vi "Post VI Refnum.vi"(8 "error in (no error)":errorcluster, 11 "Controller Template in":refnum<class "DemoCameraController.lvclass">) -> (0 "error out":errorcluster, 3 "Controller Template out":refnum<class "DemoCameraController.lvclass">)   [LabVIEW 2020, in "DemoCameraController.lvlib" / "DemoCameraController.lvclass"]
uses:
  DemoCameraController.lvclass
  C:/Program Files/National Instruments/LabVIEW 2020/vi.lib/ActorFramework/Actor/Actor.lvclass
  <vilib>/ActorFramework/Actor/Actor.lvclass/Actor.ctl
  DemoCameraController.lvclass/DemoCameraController.ctl
  Model/Hardware Abstraction Layer/Component/Device/Device Messages/Post VI Refnum Msg/Post VI Refnum Msg.lvclass/Post VI Refnum Msg.ctl
  <vilib>/ActorFramework/Message Enqueuer/Message Enqueuer.lvclass/Message Enqueuer.ctl
  <vilib>/ActorFramework/Message Enqueuer/Enqueue.vi
  Model/Hardware Abstraction Layer/Component/Device/Device Messages/Post VI Refnum Msg/Post VI Refnum Msg.lvclass
  C:/Program Files/National Instruments/LabVIEW 2020/vi.lib/ActorFramework/Message/Message.lvclass
  <vilib>/ActorFramework/Message Priority Queue/Priority Enqueue.vi
  <vilib>/ActorFramework/Actor/Actor.lvclass
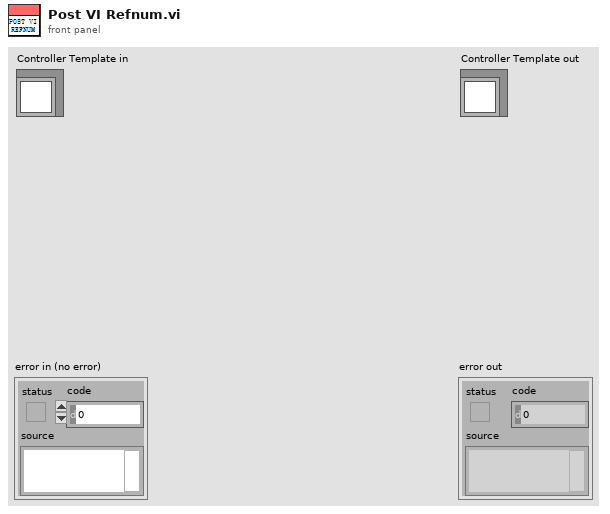
[diagram p1: front panel]
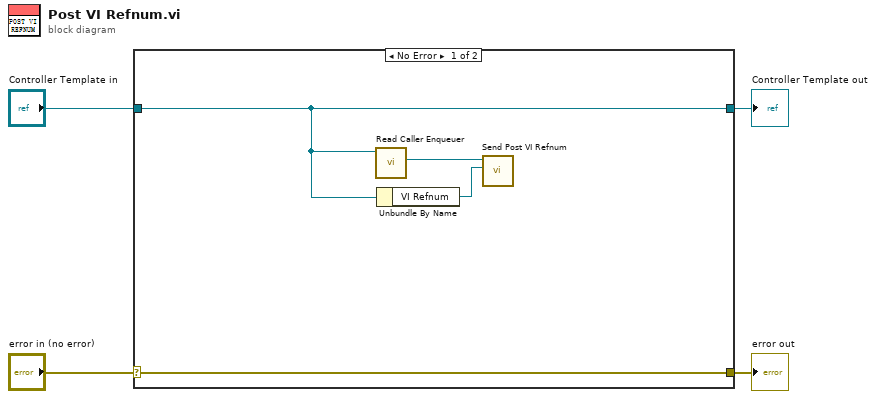
[diagram p0: block diagram]
diagram:
  n1 = case shown="No Error" "error in (no error)" {
    selector: "error in (no error)" -> [w8 w10]
    tunnel: [w8 w10] -> w3
    tunnel: [w5 w9] -> w1
    tunnel: "Controller Template in" -> [w5 w9]
    frame No Error {
      n2 = call <vilib>:"Read Caller Enqueuer.vi"("Actor"=w5) -> ("Caller Enqueuer"=w7:refnum<class "Message Enqueuer.lvclass">)  [unwired: 10 in]
      n3 = Unbundle By Name(w5) -> ("VI Refnum"=w6:refnum<vi>)
      n4 = call "Send Post VI Refnum.vi"("VI Refnum"=w6, "Message Enqueuer"=w7) -> ()  [unwired: 8 in, 2 out]
    }
    frame Error {
    }
  }
  "error out" <- w3
  "Controller Template out" <- w1
